vi "autoqueue_dynamic.vi"(0 "cluster":T5, 1 "1to4":T3, 3 "path?":bool, 4 "xy dynamic array":T1(array[cluster]), 5 "error out":errorcluster, 6 "output cluster":T4, 7 "reference":refnum<vi>, 9 "index":dbl, 10 "last time":dbl, 11 "Str Refnum":refnum<vi>, 12 "Cluster":cluster{"1":bool, "2":bool}, 13 "reference 2":refnum<vi>, 14 "Report Data.Degree":dbl[][](array[numeric]), 15 "milliseconds to wait":u32=100, 17 "milliseconds to wait 2":u32=100) -> (19 "error out 2":errorcluster)   [LabVIEW 2015]
uses:
  Typedef/Inst. Queue.ctl
  Typedef/State.ctl
panel:
  in  "Array  1":T2(array[cluster])
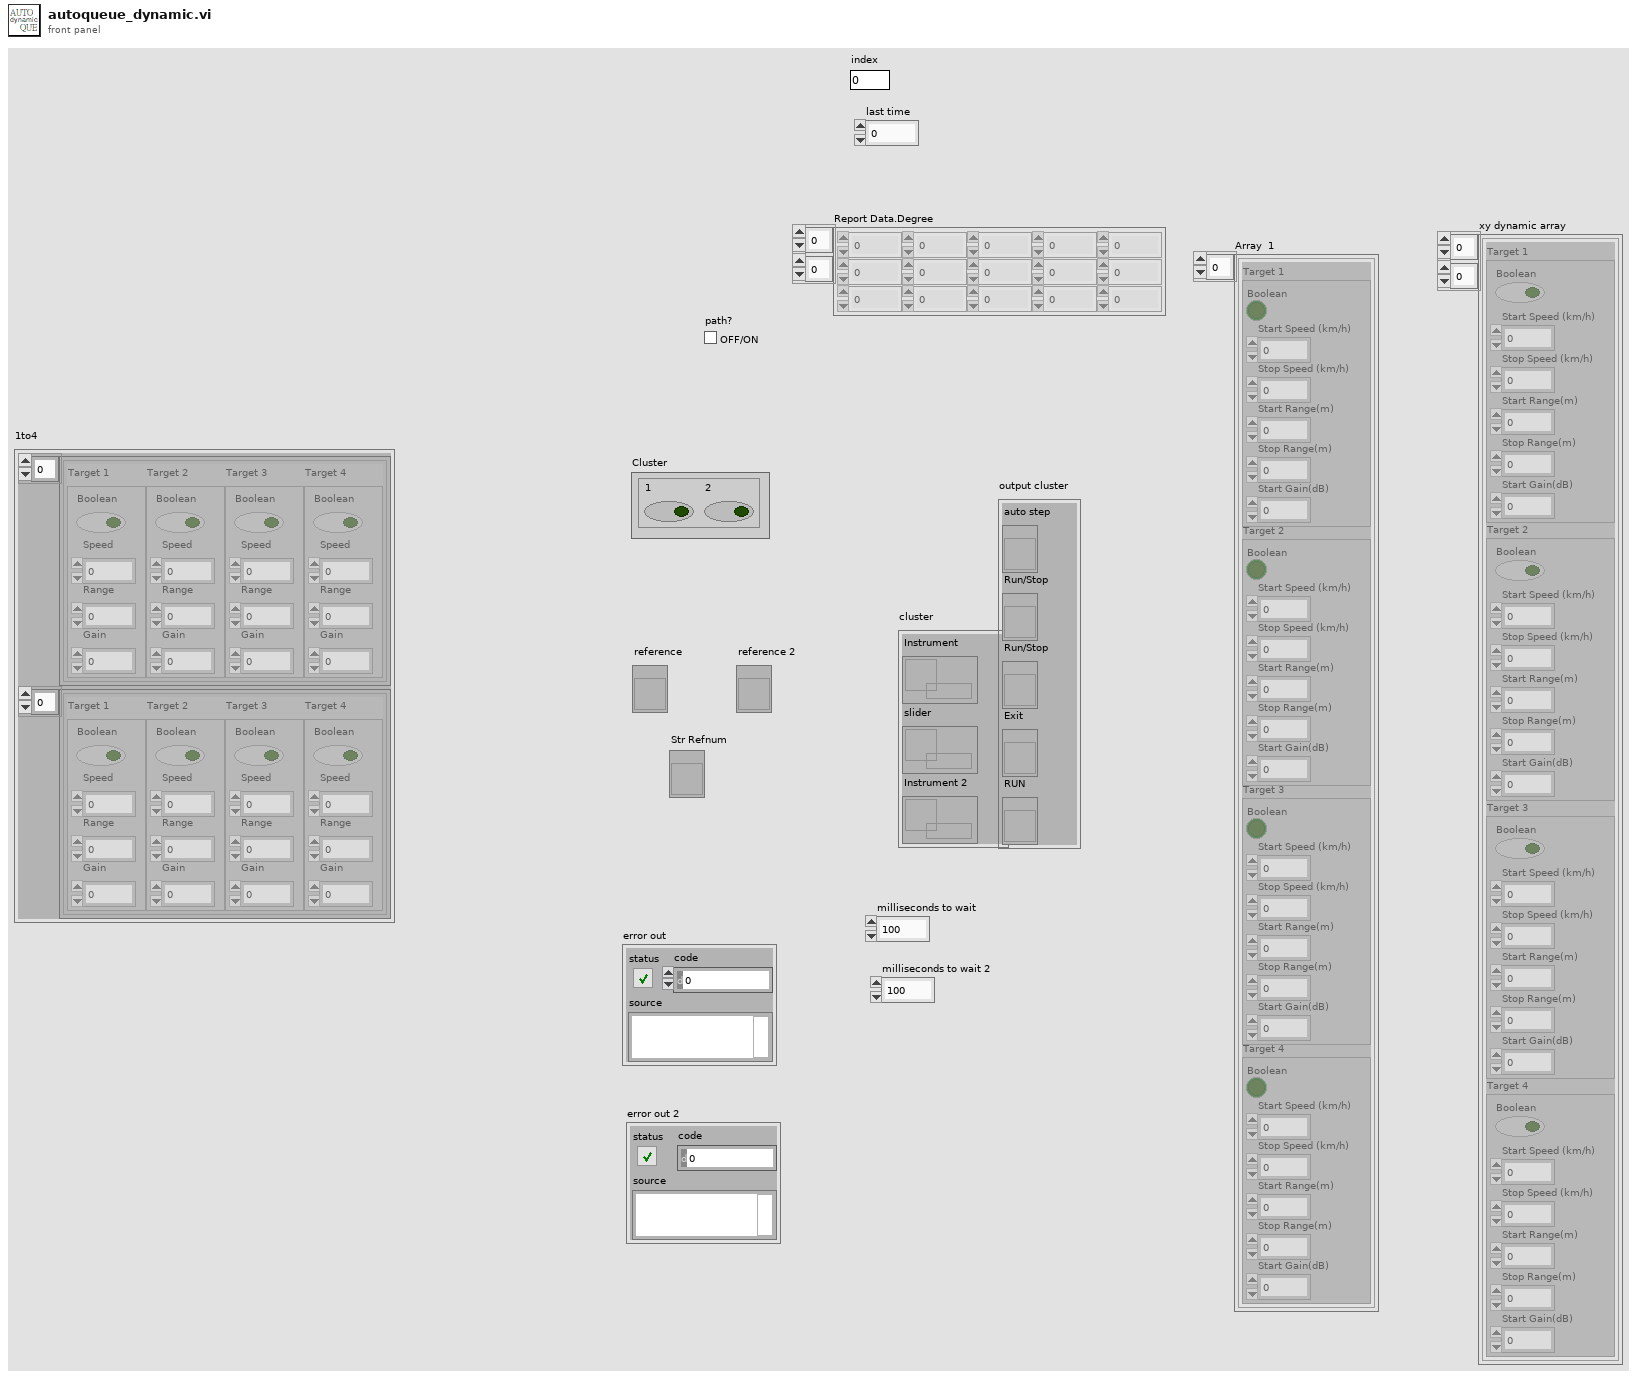
[diagram p1: front panel]
types:
  T1 = cluster{"Target 1":cluster{"Boolean":bool, "Start Speed (km/h)":dbl, "Stop Speed (km/h)":dbl, "Start Range(m)":dbl, "Stop Range(m)":dbl, "Start Gain(dB)":dbl}, "Target 2":cluster{"Boolean":bool, "Start Speed (km/h)":dbl, "Stop Speed (km/h)":dbl, "Start Range(m)":dbl, "Stop Range(m)":dbl, "Start Gain(dB)":dbl}, "Target 3":cluster{"Boolean":bool, "Start Speed (km/h)":dbl, "Stop Speed (km/h)":dbl, "Start Range(m)":dbl, "Stop Range(m)":dbl, "Start Gain(dB)":dbl}, "Target 4":cluster{"Boolean":bool, "Start Speed (km/h)":dbl, "Stop Speed (km/h)":dbl, "Start Range(m)":dbl, "Stop Range(m)":dbl, "Start Gain(dB)":dbl}}[][]
  T2 = cluster{"Target 1":cluster{"Boolean":bool, "Start Speed (km/h)":dbl, "Stop Speed (km/h)":dbl, "Start Range(m)":dbl, "Stop Range(m)":dbl, "Start Gain(dB)":dbl}, "Target 2":cluster{"Boolean":bool, "Start Speed (km/h)":dbl, "Stop Speed (km/h)":dbl, "Start Range(m)":dbl, "Stop Range(m)":dbl, "Start Gain(dB)":dbl}, "Target 3":cluster{"Boolean":bool, "Start Speed (km/h)":dbl, "Stop Speed (km/h)":dbl, "Start Range(m)":dbl, "Stop Range(m)":dbl, "Start Gain(dB)":dbl}, "Target 4":cluster{"Boolean":bool, "Start Speed (km/h)":dbl, "Stop Speed (km/h)":dbl, "Start Range(m)":dbl, "Stop Range(m)":dbl, "Start Gain(dB)":dbl}}[]
  T3 = cluster{cluster{"Target 1":cluster{"Boolean":bool, "Speed":dbl, "Range":dbl, "Gain":dbl}, "Target 2":cluster{"Boolean":bool, "Speed":dbl, "Range":dbl, "Gain":dbl}, "Target 3":cluster{"Boolean":bool, "Speed":dbl, "Range":dbl, "Gain":dbl}, "Target 4":cluster{"Boolean":bool, "Speed":dbl, "Range":dbl, "Gain":dbl}}[], cluster{"Target 1":cluster{"Boolean":bool, "Speed":dbl, "Range":dbl, "Gain":dbl}, "Target 2":cluster{"Boolean":bool, "Speed":dbl, "Range":dbl, "Gain":dbl}, "Target 3":cluster{"Boolean":bool, "Speed":dbl, "Range":dbl, "Gain":dbl}, "Target 4":cluster{"Boolean":bool, "Speed":dbl, "Range":dbl, "Gain":dbl}}[]}
  T4 = cluster{"auto step":refnum<vi>, "Run/Stop":refnum<vi>, "Run/Stop":refnum<vi>, "Exit":refnum<vi>, "RUN":refnum<vi>}
  T5 = cluster{"Instrument":refnum<queue>, "slider":refnum<queue>, "Instrument 2":refnum<queue>}
  T6 = typedef "Inst. Queue.ctl" = cluster{enum16{"auto mode", "Idle", "Inst. Connect", "£m Data", "Inst. Update", "Freq. (GHz)", "rx att", "GTX (dB)", "GRX (dB)", "Range Trim(m)", "Gain Trim (dB)", "Distance to RUT", "Mapping", "Convert", "RF ON/OFF", "Run", "Direct Program", "Stop", "Dynamic", "dyset", "Exit"}, "variant":variant}
  T7 = typedef "State.ctl" = enum16{"Idle", "Initial", "Update", "get angle", "Axis", "Connect", "Creep", "Speed", "Distance", "Move Method", "Move Mode", "Direct of Movement", "Initail Speed", "Sramp", "Normal Open", "Acceleration", "Deceleration", "Angle", "Move&Rotate", "Rotate", "Rotate_2", "Return to Origin", "Move", "Inching", "Return to Zero", "Return to Middle", "Go to Step1", "Go to Step2", "Go to Step3", "Initial to Y Step", "Select Speed", "auto mode", "Stop", "reset xy", "reset ant", "set speed", "Exit"}
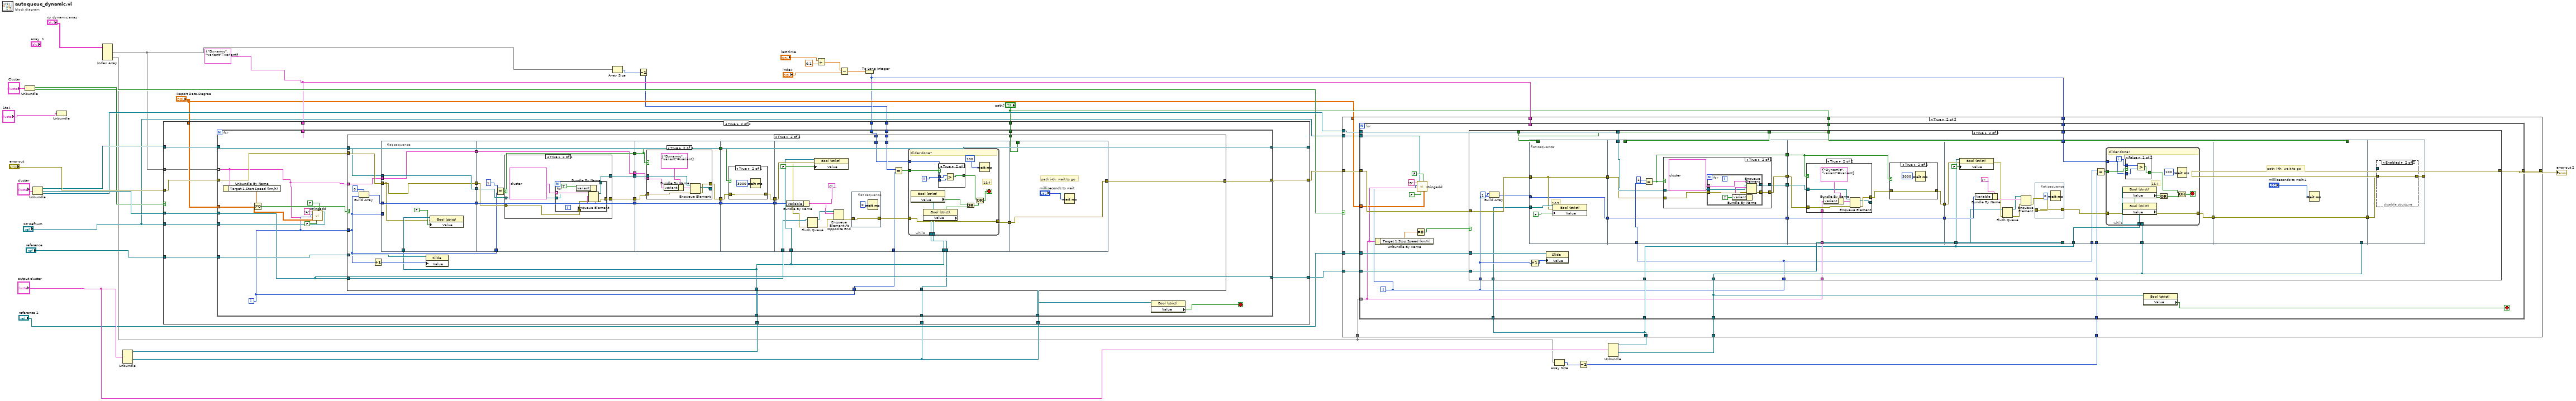
[diagram p0: block diagram]
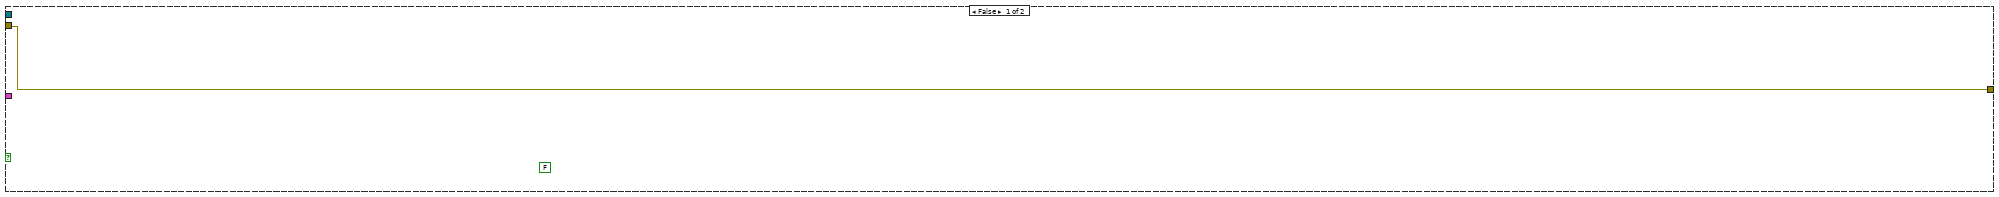
[diagram p3: hidden frame]
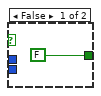
[diagram p7: hidden frame]
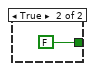
[diagram p13: hidden frame]
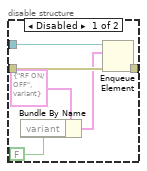
[diagram p14: hidden frame]
diagram:
  w17 = T6 {enum."Dynamic", "variant"=variant}
  n1 = Unbundle("Cluster") -> ("1"=w19:bool, "2"=w18:bool)
  n2 = Unbundle("cluster") -> ("Instrument"=w34:refnum<queue>, "slider"=w33:refnum<queue>, "Instrument 2"=w25:refnum<queue>)
  n3 = Unbundle("1to4") -> ()  [unwired: 2 out]
  n4 = Index Array(array="xy dynamic array") -> (element #1=w7:T2, element #2=w6:T2)  [unwired: 4 in]
  n5 = Unbundle("output cluster") -> ("auto step"=w23:refnum<vi>, "Exit"=w22:refnum<vi>)  [unwired: 3 out]
  n6 = Array Size(array=w7) -> (size(s)=w4:i32)
  n7 = Decrement(x=w4) -> (x-1=w3:i32)
  n8 = Divide(x="last time", y=0.1) -> (x/y=w10:dbl)
  n9 = Subtract(x=w10, y="index") -> (x-y=w8:dbl)
  n10 = To Long Integer(number=w8) -> (32bit integer=w5:i32)
  n11 = case shown="True" w19 {
    tunnel: "error out" -> [w39 w56]
    tunnel: w34 -> [w38 w55]
    tunnel: w33 -> [w37 w54]
    tunnel: [w39 w53] -> w32
    tunnel: "reference" -> [_ w52]
    tunnel: [w38 w51] -> _
    tunnel: [w37 w50] -> w27
    tunnel: w23 -> [_ w49]
    tunnel: w22 -> [_ w48]
    tunnel: w22 -> [_ w47]
    tunnel: w17 -> [_ w46]
    tunnel: "Str Refnum" -> [_ w45]
    tunnel: "path?" -> [_ w44]
    tunnel: "Report Data.Degree" -> [_ w43]
    tunnel: w7 -> [_ w42]
    tunnel: w3 -> [_ w41]
    tunnel: w5 -> [_ w40]
    frame False {
    }
    frame True {
      n12 = for {
        tunnel: w55 -> [w74]
        tunnel: w54 -> [w73]
        tunnel: w52 -> [w75]
        tunnel: [w74] -> w51
        tunnel: [w73] -> w50
        tunnel: w49 -> [w69]
        tunnel: w48 -> [w72]
        tunnel: w47 -> [w71]
        tunnel: w46 -> [_]
        tunnel: w45 -> [w63]
        tunnel: w56 -> [w76]
        tunnel: [w77] -> w53
        tunnel: w44 -> [w68]
        tunnel: w43 -> [w61]
        tunnel: w42 -> [w59] mode=indexing
        tunnel: w41 -> [w58]
        tunnel: w40 -> [w57]
        i -> [w60]
        stop <- w70 stop-if-true
        n13 = Unbundle By Name(w59) -> ("Target 1.Start Speed (km/h)"=w67:dbl)
        n14 = Not Equal To 0?(x=w67) -> (x != 0?=w66:bool)
        n15 = call "stringadd.vi"("Report Data.Degree"=w61, "Mode"=FALSE, "s/d setting"=FALSE, "Str Refnum"=w63, "variant"=w59, "Numeric"=w60, "String"="A") -> ()  [unwired: 5 in]
        n16 = case shown="True" w66 {
          tunnel: [w78 w97] -> w77
          tunnel: w76 -> [w78 w109]
          tunnel: w75 -> [_ w108]
          tunnel: w74 -> [_ w107]
          tunnel: w73 -> [_ w106]
          tunnel: w72 -> [_ w102]
          tunnel: w60 -> [_ w95]
          tunnel: w69 -> [_ w82]
          tunnel: w68 -> [_ w101]
          tunnel: w59 -> [_ w105]
          tunnel: w60 -> [_ w80]
          tunnel: w58 -> [_ w81]
          tunnel: w57 -> [_ w79]
          frame False {
            (unwired) FALSE ("Value")
          }
          frame True {
            n17 = Build Array(0 ("element"), w95) -> (w96:i32[])
            n18 = Increment(x=w95) -> (x+1=w104:i32)
            n19 = flat-sequence {
              tunnel: w96 -> [w115]
              tunnel: w109 -> [w110]
              tunnel: w107 -> [w112]
              tunnel: w105 -> [w111]
              tunnel: [w115] -> w100
              tunnel: w82 -> [w114]
              tunnel: [w110] -> w99
              tunnel: w95 -> [_]
              tunnel: [w112] -> w90
              tunnel: [w111] -> w88
              tunnel: w100 -> [w124]
              tunnel: [w124] -> w94
              tunnel: w99 -> [w123]
              tunnel: [w122] -> w93
              tunnel: w95 -> [w120]
              tunnel: [w119] -> w92
              tunnel: [w118] -> w91
              tunnel: w90 -> [w121]
              tunnel: [w117] -> w89
              tunnel: w88 -> [w117]
              tunnel: w94 -> [w144]
              tunnel: [w144] -> w87
              tunnel: w93 -> [w141]
              tunnel: [w140] -> w85
              tunnel: w92 -> [w143]
              tunnel: w91 -> [w139]
              tunnel: w89 -> [w142]
              tunnel: [w139] -> w83
              tunnel: w87 -> [w157]
              tunnel: [w157] -> w86
              tunnel: w85 -> [w156]
              tunnel: [w155] -> w84
              tunnel: w83 -> [w154]
              tunnel: w106 -> [w168]
              tunnel: w86 -> [w178]
              tunnel: w82 -> [w176]
              tunnel: w102 -> [w175]
              tunnel: [w174] -> w98
              tunnel: w84 -> [w171]
              tunnel: w82 -> [w170]
              tunnel: w81 -> [w164]
              tunnel: w80 -> [w163]
              tunnel: w79 -> [w161]
              tunnel: w101 -> [_]
              tunnel: w98 -> [w199]
              tunnel: [w199] -> w97
              frame #0 {
                n20 = property on="Property Node" class="Bool (strict)"(reference=w114, error in=w110, "Value"=FALSE) -> ()  [unwired: 2 out]
              }
              frame #1 {
                n21 = Equal?(x=1 ("element"), y=w120) -> (x = y?=w118:bool)
                n22 = case shown="True" w118 {
                  tunnel: [w126 w131] -> w122
                  tunnel: w123 -> [w126 w130]
                  tunnel: w121 -> [w125 w129]
                  tunnel: [w125 w127] -> w119
                  frame False {
                  }
                  frame True {
                    n23 = for {
                      tunnel: T6[] [{enum."Convert", "variant"=variant}, {enum."RF ON/OFF", "variant"=variant}] -> [w137] mode=indexing
                      tunnel: [w138] -> w131
                      tunnel: w130 -> [w134]
                      tunnel: w129 -> [w133]
                      tunnel: [w132] -> w127
                      n24 = Bundle By Name(cluster=w137, "variant"=TRUE) -> (w136:T6)
                      n25 = Enqueue Element(queue=w133, element=w136, error in (no error)=w134) -> (queue out=w132:refnum<queue>, error out=w138:errorcluster)  [unwired: 1 in, 1 out]
                    }
                  }
                }
              }
              frame #2 {
                n26 = case shown="True" w139 {
                  tunnel: [w146 w152] -> w140
                  tunnel: w142 -> [_ w151]
                  tunnel: w143 -> [w145 w149]
                  tunnel: [w145 w148] -> _
                  tunnel: w141 -> [w146 w147]
                  frame False {
                  }
                  frame True {
                    n27 = Bundle By Name(cluster=T6 {enum."Dynamic", "variant"=variant}, "variant"=w151) -> (w153:T6)
                    n28 = Enqueue Element(queue=w149, element=w153, error in (no error)=w147) -> (queue out=w148:refnum<queue>, error out=w152:errorcluster)  [unwired: 1 in, 1 out]
                  }
                }
              }
              frame #3 {
                n29 = case shown="True" w154 {
                  tunnel: w156 -> [w158 w160]
                  tunnel: [w158 w160] -> w155
                  frame False {
                  }
                  frame True {
                    n30 = Wait (ms)(milliseconds to wait=u32 3000) -> ()  [unwired: 1 out]
                  }
                }
              }
              frame #4 {
                n31 = Bundle By Name(cluster=cluster{"State":T7, "Variable":variant} {"State"=enum."auto mode", "Variable"=variant}, "Variable"=w178) -> (w177:cluster{"State":T7, "Variable":variant})
                n32 = property class="Bool (strict)"(reference=w170, error in=w171, "Value"=FALSE) -> (error out=w165:errorcluster)  [unwired: 1 out]
                n33 = Flush Queue(queue=w168, error in (no error)=w165) -> (queue out=w167:refnum<queue>, error out=w166:errorcluster)  [unwired: 1 out]
                n34 = Enqueue Element At Opposite End(queue=w167, element=w177, error in (no error)=w166) -> (error out=w173:errorcluster)  [unwired: 1 in, 2 out]
                n35 = flat-sequence {
                  tunnel: w173 -> [w181]
                  tunnel: [w181] -> w172
                  frame #0 {
                    n36 = Wait (ms)(milliseconds to wait=u32 0) -> ()  [unwired: 1 out]
                  }
                }
                n37 = Equal?(x=w164, y=w163) -> (x = y?=w162:bool)
                n38 = while {
                  tunnel: [w188] -> w174
                  tunnel: w175 -> [w190]
                  tunnel: w176 -> [w189]
                  tunnel: w172 -> [w188]
                  tunnel: w162 -> [w187]
                  tunnel: w161 -> [w183]
                  i -> [w182]
                  stop <- w185 stop-if-true
                  # "1&4"
                  # "slider done?"
                  n39 = property on="Property Node" class="Bool (strict)"(reference=w190) -> ("Value"=w192:bool)  [unwired: 1 in, 2 out]
                  n40 = property on="Property Node" class="Bool (strict)"(reference=w189) -> ("Value"=w191:bool)  [unwired: 1 in, 2 out]
                  n41 = case shown="True" w187 {
                    tunnel: [FALSE w197] -> w184
                    tunnel: w183 -> [_ w195]
                    tunnel: w182 -> [_ w196]
                    frame False {
                    }
                    frame True {
                      n42 = Greater?(x=w196, y=w195) -> (0:w197:bool)
                    }
                  }
                  n43 = Or(x=w192, y=w191) -> (x .or. y?=w186:bool)
                  n44 = Or(x=w184, y=w186) -> (x .or. y?=w185:bool)
                  n45 = Wait (ms)(milliseconds to wait=u32 100) -> ()  [unwired: 1 out]
                }
              }
              frame #5 {
                # "path i-th  wait to go"
                n46 = Wait (ms)(milliseconds to wait="milliseconds to wait") -> ()  [unwired: 1 out]
              }
            }
            n47 = property class="Slide"(reference=w108, "Value"=w104) -> ()  [unwired: 1 in, 2 out]
          }
        }
        n48 = property on="Property Node" class="Bool (strict)"(reference=w71) -> ("Value"=w70:bool)  [unwired: 1 in, 2 out]
      }
    }
  }
  n49 = Array Size(array=w6) -> (size(s)=w2:i32)
  n50 = Decrement(x=w2) -> (x-1=w1:i32)
  n51 = Unbundle("output cluster") -> ("auto step"=w21:refnum<vi>, "Exit"=w20:refnum<vi>)  [unwired: 3 out]
  n52 = case shown="True" w18 {
    tunnel: w32 -> [w200 w214]
    tunnel: [w200 w213] -> w31
    tunnel: "reference 2" -> [_ w212]
    tunnel: w25 -> [_ w211]
    tunnel: w27 -> [_ w210]
    tunnel: w21 -> [_ w205]
    tunnel: w20 -> [_ w209]
    tunnel: w17 -> [_ w208]
    tunnel: "path?" -> [_ w207]
    tunnel: "Report Data.Degree" -> [_ w206]
    tunnel: w6 -> [_ w204]
    tunnel: "Str Refnum" -> [_ w203]
    tunnel: w1 -> [_ w202]
    tunnel: w5 -> [_ w201]
    frame False {
    }
    frame True {
      n53 = for {
        tunnel: w212 -> [w233]
        tunnel: w211 -> [w231]
        tunnel: w210 -> [w232]
        tunnel: w205 -> [w229]
        tunnel: w209 -> [w228]
        tunnel: w208 -> [_]
        tunnel: w214 -> [w234]
        tunnel: [w235] -> w213
        tunnel: w207 -> [w225]
        tunnel: w206 -> [w220]
        tunnel: w205 -> [w224]
        tunnel: w204 -> [w219] mode=indexing
        tunnel: w203 -> [w217]
        tunnel: w202 -> [w216]
        tunnel: w201 -> [w215]
        i -> [w218]
        stop <- w230 stop-if-true
        n54 = Unbundle By Name(w219) -> ("Target 1.Stop Speed (km/h)"=w227:dbl)
        n55 = Not Equal To 0?(x=w227) -> (x != 0?=w226:bool)
        n56 = call "stringadd.vi"("Report Data.Degree"=w220, "Mode"=FALSE, "s/d setting"=FALSE, "Str Refnum"=w217, "variant"=w219, "Numeric"=w218, "String"="B") -> ()  [unwired: 5 in]
        n57 = case shown="True" w226 {
          tunnel: [w236 w265] -> w235
          tunnel: w234 -> [w236 w264]
          tunnel: w233 -> [_ w263]
          tunnel: w232 -> [_ w251]
          tunnel: w231 -> [_ w253]
          tunnel: w218 -> [_ w259]
          tunnel: w229 -> [_ w256]
          tunnel: w225 -> [_ w258]
          tunnel: w228 -> [_ w250]
          tunnel: w225 -> [_ w257]
          tunnel: w225 -> [_ w255]
          tunnel: w218 -> [_ w239]
          tunnel: w224 -> [_ w240]
          tunnel: w219 -> [_ w243]
          tunnel: w216 -> [_ w238]
          tunnel: w215 -> [_ w237]
          frame False {
          }
          frame True {
            n58 = Build Array(1 ("element"), w259) -> (w261:i32[])
            n59 = flat-sequence {
              tunnel: w261 -> [w266]
              tunnel: w264 -> [w267]
              tunnel: w256 -> [w269]
              tunnel: w257 -> [_]
              tunnel: [w267] -> w254
              tunnel: [w266] -> w252
              tunnel: [w277] -> w249
              tunnel: w255 -> [_]
              tunnel: w239 -> [w276]
              tunnel: w254 -> [w270]
              tunnel: w253 -> [w271]
              tunnel: w252 -> [w275]
              tunnel: [w275] -> w248
              tunnel: [w274] -> w245
              tunnel: [w272] -> w244
              tunnel: w249 -> [w297]
              tunnel: w248 -> [w298]
              tunnel: [w298] -> w247
              tunnel: [w292] -> w246
              tunnel: w245 -> [w296]
              tunnel: w244 -> [w295]
              tunnel: w243 -> [w294]
              tunnel: w247 -> [w327]
              tunnel: w251 -> [w318]
              tunnel: w250 -> [w326]
              tunnel: w240 -> [w325]
              tunnel: w246 -> [w319]
              tunnel: [w322] -> w241
              tunnel: w240 -> [w321]
              tunnel: w239 -> [w314]
              tunnel: w238 -> [w313]
              tunnel: w237 -> [w311]
              tunnel: w250 -> [_]
              tunnel: w258 -> [_]
              tunnel: [w348] -> w242
              tunnel: w241 -> [w348]
              tunnel: [w351] -> w265
              tunnel: w242 -> [w350]
              frame #0 {
                # "1&5"
                n60 = property on="Property Node" class="Bool (strict)"(reference=w269, error in=w267, "Value"=FALSE) -> ()  [unwired: 2 out]
              }
              frame #1 {
                n61 = Equal?(x=1, y=w276) -> (x = y?=w272:bool)
                n62 = case shown="True" w272 {
                  tunnel: [w279 w284] -> w277
                  tunnel: w271 -> [w278 w283]
                  tunnel: w270 -> [w279 w282]
                  tunnel: [w278 w280] -> w274
                  frame False {
                  }
                  frame True {
                    n63 = for {
                      tunnel: T6[] [{enum."Convert", "variant"=variant}, {enum."RF ON/OFF", "variant"=variant}] -> [w289] mode=indexing
                      tunnel: w282 -> [w291]
                      tunnel: [w290] -> w284
                      tunnel: w283 -> [w286]
                      tunnel: [w285] -> w280
                      n64 = Bundle By Name(cluster=w289, "variant"=TRUE) -> (w288:T6)
                      n65 = Enqueue Element(queue=w286, element=w288, error in (no error)=w291) -> (queue out=w285:refnum<queue>, error out=w290:errorcluster)  [unwired: 1 in, 1 out]
                    }
                  }
                }
              }
              frame #2 {
                n66 = case shown="True" w295 {
                  tunnel: [w303 w309] -> w293
                  tunnel: w296 -> [w302 w307]
                  tunnel: [w302 w306] -> _
                  tunnel: w297 -> [w303 w305]
                  tunnel: w294 -> [_ w304]
                  frame False {
                  }
                  frame True {
                    n67 = Bundle By Name(cluster=T6 {enum."Dynamic", "variant"=variant}, "variant"=w304) -> (w310:T6)
                    n68 = Enqueue Element(queue=w307, element=w310, error in (no error)=w305) -> (queue out=w306:refnum<queue>, error out=w309:errorcluster)  [unwired: 1 in, 1 out]
                  }
                }
                n69 = case shown="True" w295 {
                  tunnel: w293 -> [w299 w300]
                  tunnel: [w299 w300] -> w292
                  frame False {
                  }
                  frame True {
                    n70 = Wait (ms)(milliseconds to wait=u32 3000) -> ()  [unwired: 1 out]
                  }
                }
              }
              frame #3 {
                n71 = property class="Bool (strict)"(reference=w321, error in=w319, "Value"=FALSE) -> (error out=w315:errorcluster)  [unwired: 1 out]
                n72 = Bundle By Name(cluster=cluster{"State":T7, "Variable":variant} {"State"=enum."auto mode", "Variable"=variant}, "Variable"=w327) -> (w329:cluster{"State":T7, "Variable":variant})
                n73 = Flush Queue(queue=w318, error in (no error)=w315) -> (queue out=w317:refnum<queue>, error out=w316:errorcluster)  [unwired: 1 out]
                n74 = Enqueue Element(queue=w317, element=w329, error in (no error)=w316) -> (error out=w324:errorcluster)  [unwired: 1 in, 2 out]
                n75 = flat-sequence {
                  tunnel: w324 -> [w331]
                  tunnel: [w331] -> w323
                  frame #0 {
                    n76 = Wait (ms)(milliseconds to wait=u32 0) -> ()  [unwired: 1 out]
                  }
                }
                n77 = Equal?(x=w314, y=w313) -> (x = y?=w312:bool)
                n78 = while {
                  tunnel: w323 -> [w343]
                  tunnel: [w343] -> w322
                  tunnel: w326 -> [w339]
                  tunnel: w325 -> [w338]
                  tunnel: w312 -> [w335]
                  tunnel: w311 -> [w333]
                  i -> [w332]
                  stop <- w337 stop-if-true
                  # "1&4"
                  # "slider done?"
                  n79 = property on="Property Node" class="Bool (strict)"(reference=w339) -> ("Value"=w341:bool)  [unwired: 1 in, 2 out]
                  n80 = property on="Property Node" class="Bool (strict)"(reference=w338) -> ("Value"=w340:bool)  [unwired: 1 in, 2 out]
                  n81 = case shown="False" w335 {
                    tunnel: [w344 FALSE] -> w334
                    tunnel: w333 -> [w345 _]
                    tunnel: w332 -> [w346 _]
                    frame False {
                      n82 = Greater?(x=w346, y=w345) -> (0:w344:bool)
                    }
                    frame True {
                    }
                  }
                  n83 = Or(x=w341, y=w340) -> (x .or. y?=w336:bool)
                  n84 = Wait (ms)(milliseconds to wait=u32 100) -> ()  [unwired: 1 out]
                  n85 = Or(x=w334, y=w336) -> (x .or. y?=w337:bool)
                }
              }
              frame #4 {
                # "path i-th  wait to go"
                n86 = Wait (ms)(milliseconds to wait="milliseconds to wait 2") -> ()  [unwired: 1 out]
              }
              frame #5 {
                n87 = disable-structure shown="Enabled" {
                  disable-tunnel: [w357 w358] -> w351
                  disable-tunnel: w350 -> [w356 w358]
                  disable-tunnel: _ -> [w352 _]
                  frame Disabled {
                    n88 = Bundle By Name(cluster=T6 {enum."RF ON/OFF", "variant"=variant}, "variant"=FALSE) -> (w354:T6)
                    n89 = Enqueue Element(queue=w352, element=w354, error in (no error)=w356) -> (error out=w357:errorcluster)  [unwired: 1 in, 2 out]
                  }
                  frame Enabled {
                  }
                }
              }
            }
            n90 = Increment(x=w259) -> (x+1=w262:i32)
            n91 = property class="Slide"(reference=w263, "Value"=w262) -> ()  [unwired: 1 in, 2 out]
          }
        }
        n92 = property on="Property Node" class="Bool (strict)"(reference=w228) -> ("Value"=w230:bool)  [unwired: 1 in, 2 out]
      }
    }
  }
  "error out 2" <- w31
